vi "SetHostBooleanFlags.vi"(0 "reference":refnum<vi>, 5 "Control Name":string="clear err", 7 "Boolean":bool=TRUE) -> (4 "reference out":refnum<vi>, 15 "error out":errorcluster)   [LabVIEW 2019]
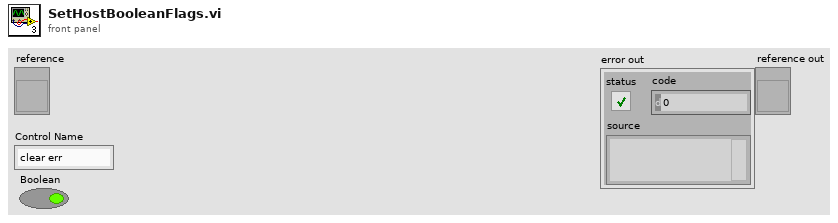
[diagram p1: front panel]
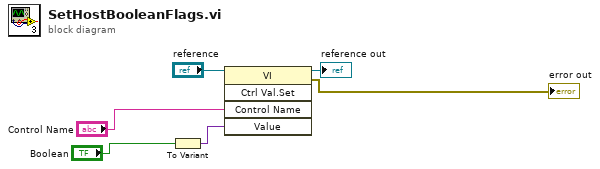
[diagram p0: block diagram]
diagram:
  n1 = To Variant(anything="Boolean") -> (Variant=w3:variant)
  n2 = invoke class="VI" method="Ctrl Val.Set"(reference="reference", "Control Name"="Control Name", "Value"=w3) -> (reference out=→"reference out":refnum<vi>, error out=→"error out":errorcluster)  [unwired: 2 in, 3 out]
